vi "Multiply Float SCTL 40 MHz Latency 0 Pipeline 1.vi"(2 "enable":bool, 3 "y":sgl, 4 "x":sgl) -> (0 "data valid":bool, 1 "x*y":sgl)   [LabVIEW 2014]
uses:
  <vilib>/rvi/IPIntegrationNode/IPINode_Typedef/niFpgaIPINodeSupportedFamilies.ctl
  <vilib>/rvi/IPIntegrationNode/IPINode_Utilities/niFpgaIPINodeSimCore.vi
  <vilib>/rvi/XilinxIP/XIPIN_XNode/niFpgaXIPIN.xnode
  Coregen SPARTAN6/Multiply SCTL L0/Multiply_SCTL_L0_C3ADE5BE76064AA39E7EE6565DE88692.dll
  <vilib>/rvi/IPIntegrationNode/IPINode_Xnode/niFpgaIPINode.xnode
  Coregen KINTEX7/Multiply SCTL L0/xsim.dir/Multiply_SCTL_L0_91721A02967D4925A2B5FA29BCD18B30/xsimk_91721A02967D4925A2B5FA29BCD18B30.dll
  Coregen Zynq/Multiply SCTL L0/xsim.dir/Multiply_SCTL_L0_184E08AD97044BA3AD7104FB20BDBA66/xsimk_184E08AD97044BA3AD7104FB20BDBA66.dll
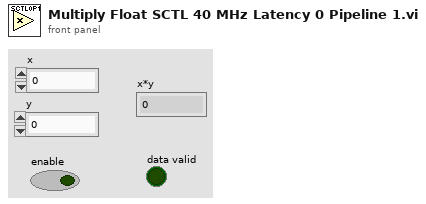
[diagram p1: front panel]
types:
  T1 = typedef "niFpgaIPINodeSupportedFamilies.ctl" = cluster{"unlimited?":bool, "supported targets":string[]}
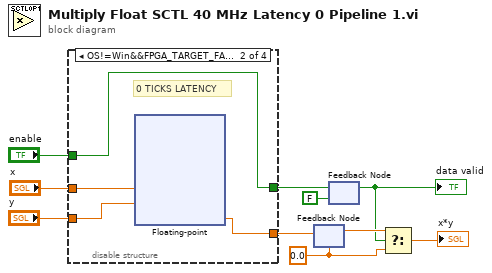
[diagram p0: block diagram]
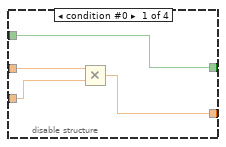
[diagram p2: hidden frame]
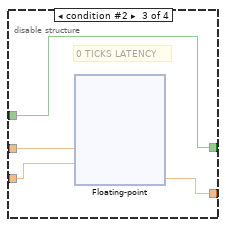
[diagram p3: hidden frame]
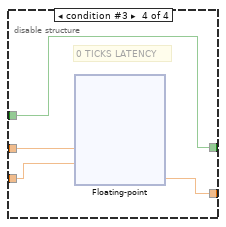
[diagram p4: hidden frame]
diagram:
  w5 = sgl 0.0 ("t")
  n1 = disable-structure shown="OS!=Win&&FPGA_TARGET_FAMILY==SPARTAN6" {
    disable-tunnel: "x" -> [w14 w18 w75 w139]
    disable-tunnel: "y" -> [w13 w17 w73 w137]
    disable-tunnel: "enable" -> [w12 w15 w76 w140]
    disable-tunnel: [w11 w16 w74 w138] -> w4
    disable-tunnel: [w12 w15 w76 w140] -> w3
    frame condition #0 {
      n2 = Multiply(x=w14, y=w13) -> (x*y=w11:sgl)
    }
    frame condition #1 (active) {
      # "0 TICKS LATENCY"
      n3 = xnode ("Floating-point")("a"=w18, "b"=w17) -> ("result"=w16:sgl)
    }
    frame condition #2 {
      # "0 TICKS LATENCY"
      n4 = xnode ("Floating-point")("s_axis_a_tdata"=w75, "s_axis_b_tdata"=w73) -> ("m_axis_result_tdata"=w74:sgl)  [unwired: 2 in, 1 out]
    }
    frame condition #3 {
      # "0 TICKS LATENCY"
      n5 = xnode ("Floating-point")("s_axis_a_tdata"=w139, "s_axis_b_tdata"=w137) -> ("m_axis_result_tdata"=w138:sgl)  [unwired: 2 in, 1 out]
    }
  }
  n6 = feedback #1(w5) -> (w7:sgl)
  n7 = feedback-in #1(w4) -> ()
  n8 = feedback #2(FALSE ("reset")) -> (w1:bool)
  "data valid" <- w1
  n9 = feedback-in #2(w3) -> ()
  n10 = Select(t=w7, s=w1, f=w5) -> (s? t:f=→"x*y":sgl)
